vi "Lookup Group.vi"(7 "Group Type (Abstract)":refnum<class "GroupAbstract.lvclass">, 8 "error in (no error)":errorcluster, 10 "Group Name":string, 11 "Task in":refnum<class "Task.lvclass">) -> (0 "error out":errorcluster, 2 "Group":refnum<class "GroupAbstract.lvclass">, 3 "Task out":refnum<class "Task.lvclass">)   [LabVIEW 2020, in "Volatus.lvlib" / "Task.lvclass"]
uses:
  Task.lvclass
  lv-vecto/Vecto/GroupAbstract/GroupAbstract.lvclass
  Task.lvclass/Task.ctl
  TelemetryAPI/TelemetryAPI.lvclass/TelemetryAPI.ctl
  TelemetryAPI/TelemetryAPI.lvclass
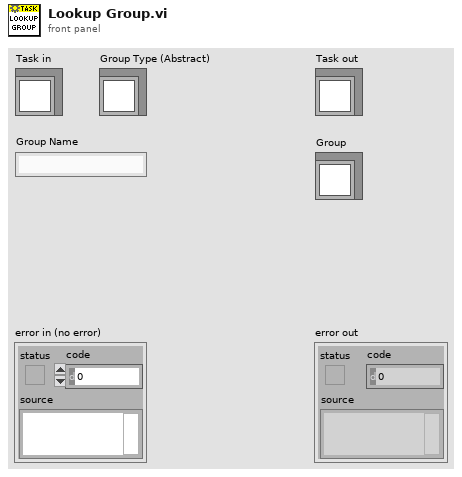
[diagram p1: front panel]
types:
  T1 = map{string, refnum<class "GroupAbstract.lvclass">}
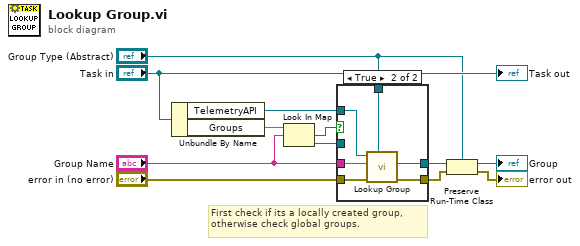
[diagram p0: block diagram]
diagram:
  # "First check if its a locally created group, otherwise check global groups."
  n1 = Unbundle By Name("Task in") -> ("TelemetryAPI"=w11:refnum<class "TelemetryAPI.lvclass">, "Groups"=w8:T1)
  n2 = Look In Map(map=w8, key="Group Name") -> (key not found?=w2:bool, value=w1:refnum<class "GroupAbstract.lvclass">)  [unwired: 1 in]
  n3 = case shown="True" w2 {
    tunnel: w11 -> [_ w20]
    tunnel: "Group Type (Abstract)" -> [_ w19]
    tunnel: [w14 w18] -> w10
    tunnel: "error in (no error)" -> [w13 w17]
    tunnel: [w13 w16] -> w5
    tunnel: "Group Name" -> [_ w15]
    tunnel: w1 -> [w14 _]
    frame False {
    }
    frame True {
      n4 = call "Lookup Group.vi"("Group Type (Abstract)"=w19, "error in (no error)"=w17, "Group Name"=w15, "TelemetryAPI in"=w20) -> ("error out"=w16:errorcluster, "Group"=w18:refnum<class "GroupAbstract.lvclass">)  [unwired: 5 in, 1 out]
    }
  }
  n5 = Preserve Run-Time Class(object in=w10, error in=w5, 2:"Group Type (Abstract)") -> (object out=→"Group":refnum<class "GroupAbstract.lvclass">, error out=→"error out":errorcluster)
  "Task out" <- "Task in"
